vi "Read ROI & calibration.vi"(8 "error in (no error)":errorcluster, 11 "Analyze BaseClass in":refnum<class "Analyze BaseClass.lvclass">) -> (0 "error out":errorcluster, 1 "ROI Descriptor":T1 {"Contours"."Type" items=["No Selection", "Point", "Line", "Rectangle", "Oval", "Polygon", "Freehand Region", "Annulus", "Unused2", "Unused3", "Broken Line", "Freehand Line", "Rotated Rectangle"]}, 2 "calibration mm/px":dbl[unit], 3 "Analyze BaseClass out":refnum<class "Analyze BaseClass.lvclass">)   [LabVIEW 2014, in "Analyze.lvlib" / "Analyze BaseClass.lvlib" / "Analyze BaseClass.lvclass"]
uses:
  Analyze BaseClass.lvclass
  Analyze Parameter/Analyze Parameter ROI/Analyze Parameter ROI.lvclass
  Analyze Parameter/Analyze Parameter Calibration/Analyze Parameter Calibration.lvclass
  Analyze Parameter/Analyze Parameter ROI/Analyze Parameter ROI.lvclass/Analyze Parameter ROI.ctl
  Analyze Parameter/Analyze Parameter Calibration/Analyze Parameter Calibration.lvclass/Analyze Parameter Calibration.ctl
  Analyze Parameter/Analyze Parameter ROI/Read ROI Descriptor.vi
  Analyze Parameter/Analyze Parameter Calibration/Read Calibration.vi
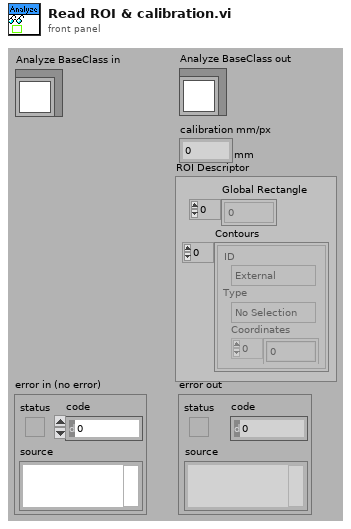
[diagram p1: front panel]
types:
  T1 = typedef "ROI Descriptor" = cluster{"Global Rectangle":i32[], "Contours":cluster{"ID":enum32{"External", "Internal"}, "Type":u32, "Coordinates":i32[]}[]}
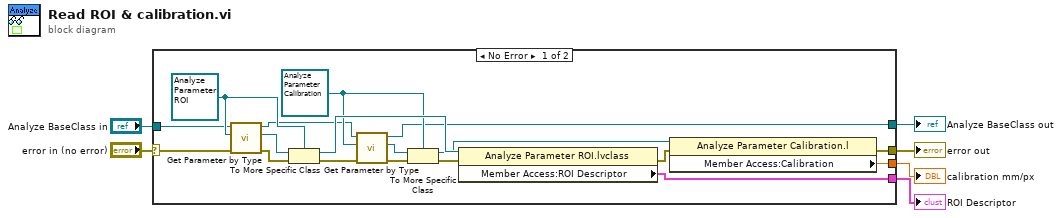
[diagram p0: block diagram]
diagram:
  n1 = case shown="No Error" "error in (no error)" {
    selector: "error in (no error)" -> [w12 w25]
    tunnel: [w7 w25] -> w5
    tunnel: [w14 w26] -> w3
    tunnel: "Analyze BaseClass in" -> [w20 w26]
    tunnel: [w24 _] -> w2
    tunnel: [w23 _] -> w1
    frame No Error {
      w18 = refnum<class "Analyze Parameter Calibration.lvclass"> refnum ("Analyze Parameter Calibration.lvclass")
      w21 = refnum<class "Analyze Parameter ROI.lvclass"> refnum ("Analyze Parameter ROI.lvclass")
      n2 = call "Get Parameter by Type.vi"("error in (no error)"=w12, "Parameter Type"=w21, "Analyze BaseClass in"=w20) -> ("error out"=w11:errorcluster, "Parameter"=w22:refnum<class "Analyze Parameter Base.lvclass">, "Analyze BaseClass out"=w15:refnum<class "Analyze BaseClass.lvclass">)  [unwired: 5 in, 1 out]
      n3 = To More Specific Class(target class=w21, reference=w22, error in=w11) -> (specific class reference=w19:refnum<class "Analyze Parameter ROI.lvclass">, error out=w10:errorcluster)
      n4 = call "Get Parameter by Type.vi"("error in (no error)"=w10, "Parameter Type"=w18, "Analyze BaseClass in"=w15) -> ("error out"=w9:errorcluster, "Parameter"=w17:refnum<class "Analyze Parameter Base.lvclass">, "Analyze BaseClass out"=w14:refnum<class "Analyze BaseClass.lvclass">)  [unwired: 5 in, 1 out]
      n5 = To More Specific Class(target class=w18, reference=w17, error in=w9) -> (specific class reference=w13:refnum<class "Analyze Parameter Calibration.lvclass">, error out=w16:errorcluster)
      n6 = property class="Analyze Parameter ROI.lvclass"(reference=w19, error in=w16) -> (error out=w8:errorcluster, "Member Access:ROI Descriptor"=w23:T1)  [unwired: 1 out]
      n7 = property class="Analyze Parameter Calibration.l"(reference=w13, error in=w8) -> (error out=w7:errorcluster, "Member Access:Calibration"=w24:dbl[unit])  [unwired: 1 out]
    }
    frame Error {
    }
  }
  "error out" <- w5
  "Analyze BaseClass out" <- w3
  "calibration mm/px" <- w2
  "ROI Descriptor" <- w1
